vi "ROIGridSize.vi"(4 "ROI Grid\nX Size":u32 caption="ROI Grid X Size", 5 "ROI Grid\nY Size":u32 caption="ROI Grid Y Size") -> (0 "OK":bool, 1 "New ROI Grid X Size":u32, 2 "New ROI Grid Y Size":u32)   [LabVIEW 2009]
panel:
  in  "OK Button":bool
  in  "Cancel Button":bool
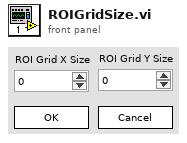
[diagram p1: front panel]
types:
  T1 = enum32{"Invalid", "Standard", "Closed", "Hidden", "Minimized", "Maximized"}
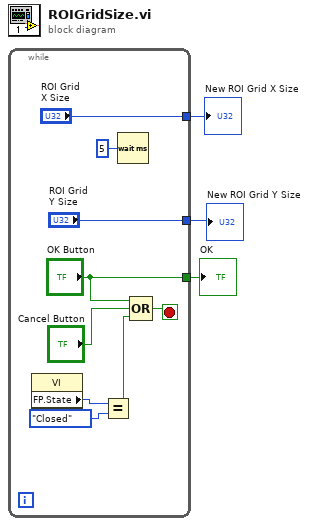
[diagram p0: block diagram]
diagram:
  n1 = while {
    tunnel: ["ROI Grid\nX Size"] -> w3
    tunnel: ["ROI Grid\nY Size"] -> w2
    tunnel: ["OK Button"] -> w1
    stop <- w10 stop-if-true
    n2 = property class="VI"() -> ("FP.State"=w7:T1)  [unwired: 2 in, 2 out]
    n3 = Equal?(x=w7, y=T1."Closed") -> (x = y?=w5:bool)
    n4 = Wait (ms)(milliseconds to wait=u32 5) -> ()  [unwired: 1 out]
    n5 = Compound Arithmetic op=OR("OK Button", "Cancel Button", w5) -> (w10:bool)
  }
  "New ROI Grid X Size" <- w3
  "New ROI Grid Y Size" <- w2
  "OK" <- w1
